vi "ErrorMngmt_CER.vi"(11 "Queue in":refnum<queue>) -> ()   [LabVIEW 2015]
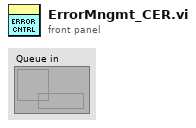
[diagram p1: front panel]
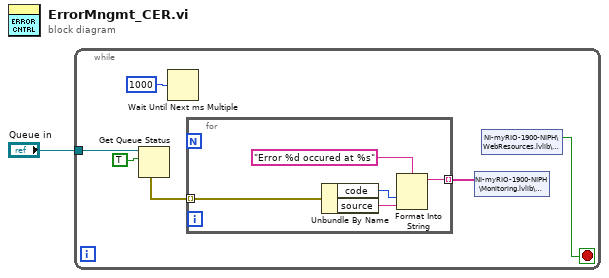
[diagram p0: block diagram]
diagram:
  n1 = while {
    tunnel: "Queue in" -> [w7]
    stop <- w2 stop-if-true
    n2 = Get Queue Status(queue=w7, return elements? (F)=TRUE) -> (elements=w5:errorcluster[])  [unwired: 1 in, 7 out]
    n3 = Wait Until Next ms Multiple(millisecond multiple=u32 1000) -> ()  [unwired: 1 out]
    n4 = for {
      tunnel: w5 -> [w12] mode=indexing
      tunnel: [w8] -> w4 mode=indexing
      n5 = Unbundle By Name(w12) -> ("code"=w11:i32, "source"=w10:string)
      n6 = Format Into String(format string="Error %d occured at %s", w11, w10) -> (resulting string=w8:string)  [unwired: 2 in, 1 out]
    }
    n7 = shared-variable "NI-myRIO-1900-NIPH\\Monitoring.lvlib\\Errors"(w4) -> ()  [unwired: 1 in, 1 out]
    n8 = shared-variable "NI-myRIO-1900-NIPH\\WebResources.lvlib\\Engine"() -> (w2:bool)  [unwired: 1 in, 1 out]
  }
